vi "Velocity-To-Dynamic.vi"(10 "Result":dbl, 11 "Waveform":waveform(dbl)) -> (3 "Dynamic Data Type":dynamicdata(waveform))   [LabVIEW 2025]
panel:
  # "Look inside LC0-To-Dynamic.vi for more information"
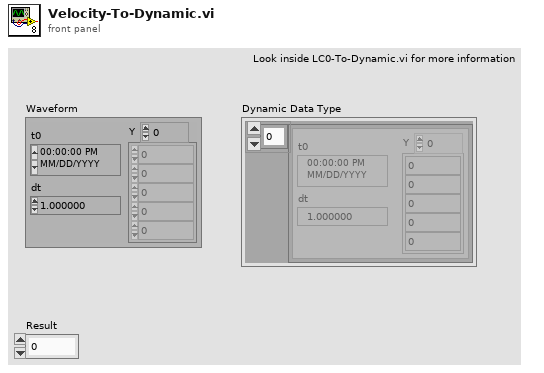
[diagram p1: front panel]
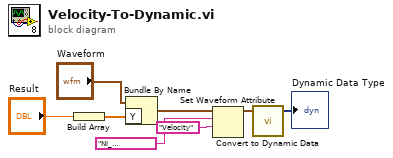
[diagram p0: block diagram]
diagram:
  n1 = Build Array("Result") -> (w2:dbl[])
  n2 = Bundle By Name(cluster="Waveform", "Y"=w2) -> (w3:waveform(dbl))
  n3 = Set Waveform Attribute(5:"Velocity", 6:"NI_ChannelName" ("name"), 7:w3) -> (3:w6:waveform(dbl))  [unwired: 1 in, 2 out]
  n4 = call "Convert to Dynamic Data"("Waveform"=w6) -> ("Dynamic Data Type"=→"Dynamic Data Type":dynamicdata)  [unwired: 3 in]
